vi "Write standard_name.vi"(8 "error in (no error)":errorcluster, 10 "standard_name":string, 11 "Pipette in":refnum<class "Pipette.lvclass">) -> (0 "error out":errorcluster, 3 "Pipette out":refnum<class "Pipette.lvclass">)   [LabVIEW 2017, in "Pipette.lvclass"]
uses:
  Pipette.lvclass
  Pipette.lvclass/Pipette.ctl
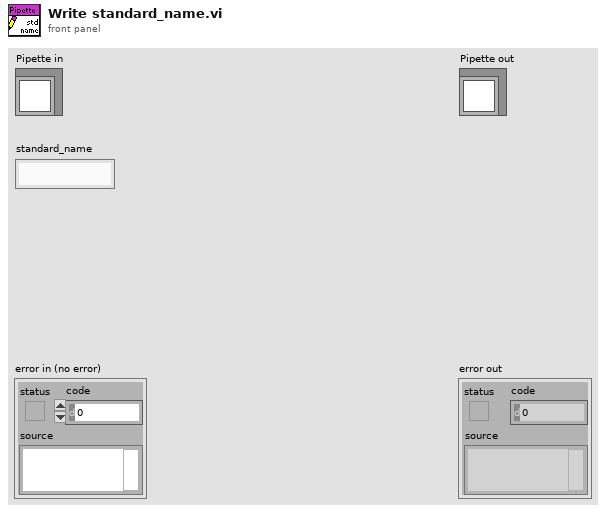
[diagram p1: front panel]
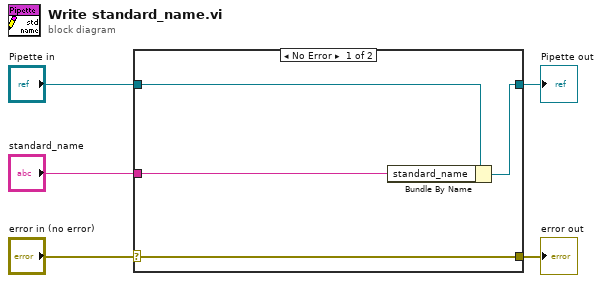
[diagram p0: block diagram]
diagram:
  n1 = case shown="No Error" "error in (no error)" {
    selector: "error in (no error)" -> [w9 w10]
    tunnel: [w9 w10] -> w4
    tunnel: [w7 w11] -> w2
    tunnel: "Pipette in" -> [w8 w11]
    tunnel: "standard_name" -> [w6 _]
    frame No Error {
      n2 = Bundle By Name(cluster=w8, "standard_name"=w6) -> (w7:refnum<class "Pipette.lvclass">)
    }
    frame Error {
    }
  }
  "error out" <- w4
  "Pipette out" <- w2
